vi "Print Number.vi"(8 "error in (no error)":errorcluster, 10 "Input":string, 11 "VISA resource name":refnum<visa-resource-name>) -> (0 "error out":errorcluster, 1 "Command String":string, 2 "Output":string, 3 "VISA resource name out":refnum<visa-resource-name>)   [LabVIEW 2018, in "Keithley 3706.lvlib"]
uses:
  <instrlib>/Keithley 3706/Keithley 3706.lvlib
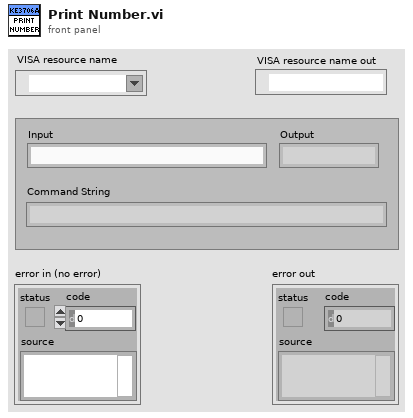
[diagram p1: front panel]
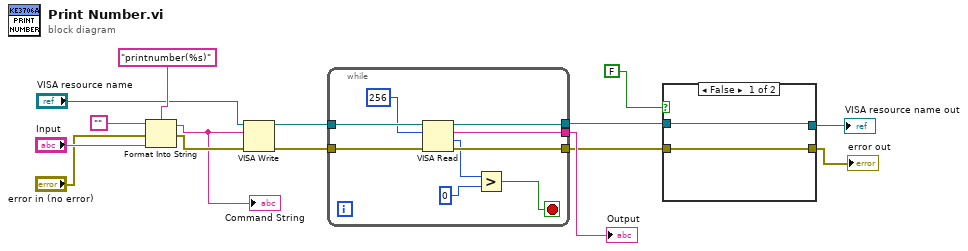
[diagram p0: block diagram]
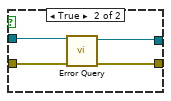
[diagram p2: hidden frame]
diagram:
  n1 = Format Into String(format string="printnumber(%s)" ("initial string"), initial string="", error in="error in (no error)", "Input") -> (resulting string=w9:string, error out=w11:errorcluster)
  "Command String" <- w9
  n2 = VISA Write(VISA resource name="VISA resource name", write buffer=w9, error in (no error)=w11) -> (VISA resource name out=w8:refnum<visa-resource-name>, error out=w7:errorcluster)  [unwired: 1 out]
  n3 = while {
    tunnel: w8 -> [w23]
    tunnel: w7 -> [w24]
    tunnel: [w22] -> w4
    tunnel: [w21] -> w3
    tunnel: [w19] -> w6
    stop <- w18 stop-if-true
    n4 = VISA Read(VISA resource name=w23, byte count=256, error in (no error)=w24) -> (VISA resource name out=w22:refnum<visa-resource-name>, read buffer=w19:string, return count=w17:u32, error out=w21:errorcluster)
    n5 = Greater?(x=w17, y=0) -> (0:w18:bool)
  }
  "Output" <- w6
  n6 = case shown="False" FALSE {
    tunnel: w4 -> [w26 w30]
    tunnel: w3 -> [w25 w29]
    tunnel: [w26 w28] -> w2
    tunnel: [w25 w27] -> w1
    frame False {
    }
    frame True {
      n7 = call <instrlib>:"Error Query.vi"("error in (no error)"=w29, "VISA resource name"=w30) -> ("error out"=w27:errorcluster, "VISA resource name output"=w28:refnum<visa-resource-name>)  [unwired: 6 in, 2 out]
    }
  }
  "VISA resource name out" <- w2
  "error out" <- w1
